vi "thermal_optical_camera_4.vi"() -> ()   [LabVIEW 2025]
uses:
  Global 1.vi
panel:
  in  "Stop (F)":bool
  in  "Acquisition Control:\nExposure Time [100, 3E7]":dbl=999.0 caption="Acquisition Control::Exposure Time" min=100.0 max=29999995.0
  in  "Analog Control:\nGain [0, 27]":dbl caption="Analog Control::Gain" min=0.0 max=27.045663671679687
  in  "Analog Control:\nBlack Level [-5, 10]":dbl caption="Analog Control::Black Level" min=-5.0000011920928955 max=10.000002384185791
  in  "Analog Control:\nGamma [0.25, 4.00]":dbl=0.800048828125 caption="Analog Control::Gamma" min=0.25 max=4.0 step=0.05
  out "Optical camera":T1(plugin-control)
  in  "optical capture interval (s)":dbl
  in  "File Path":string="C:\\Digambar\\Metal_thin_wall\\Optical_images\\Optical_images"
  out "File Name Out":string
  out "Frames":i32
  in  "thermal capture interval (s)":dbl
  out "Thermal camera":T1(plugin-control)
  out "Output":string
  in  "Flag Button":bool
  in  "Stop & Save":bool
  in  "Stop Preview":bool
  in  "Focus":dbl(slide) scale=0.0..100.0
  in  "Record":bool
  # "(1) Run VI"
  # "(2) After thermal camera calibration message (in terminal), press START"
  # "(3) Stop & Save"
  # "Destination for Optical Images:"
  # "Begin Record\nTHERMAL & OPTICAL"
  # "(Enter \"28\")"
  # "change folder names each time you run,\nso it saves data sets in dedicated folders:\nfolder1\nfolder2\nfolder3\netc..."
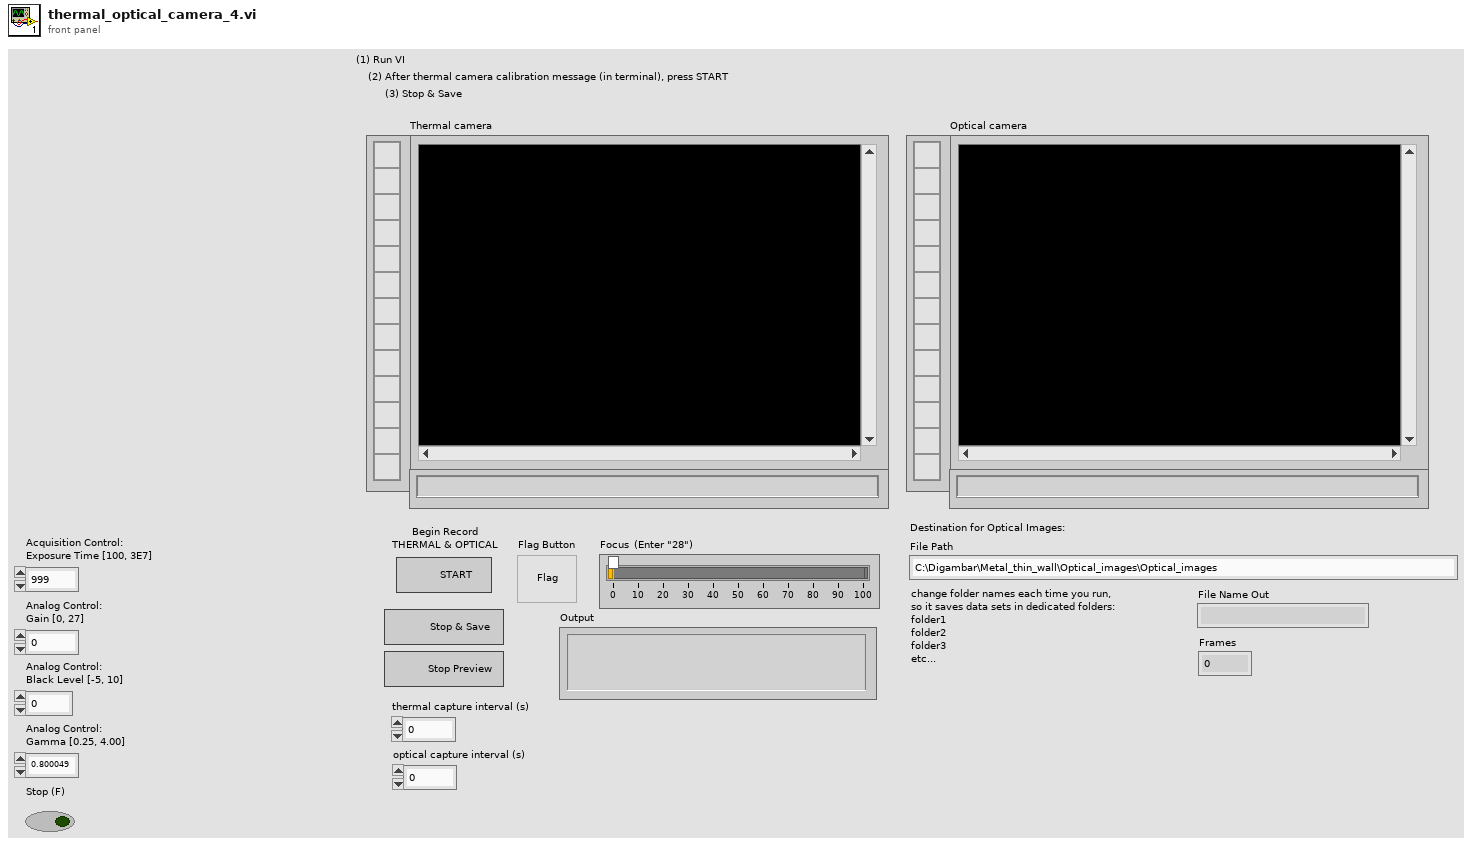
[diagram p1: front panel]
types:
  T1 = typedef "IMAQ Image.ctl" = refnum<image>
  T2 = enum16{"Standard", "Buffered", "CRLF", "Immediate"}
  T3 = enum16{"open", "replace", "create", "open or create", "replace or create", "replace or create with confirmation"}
  T4 = enum16{"big-endian, network order", "native, host order", "little-endian"}
  T5 = typedef "Image Type" = u32
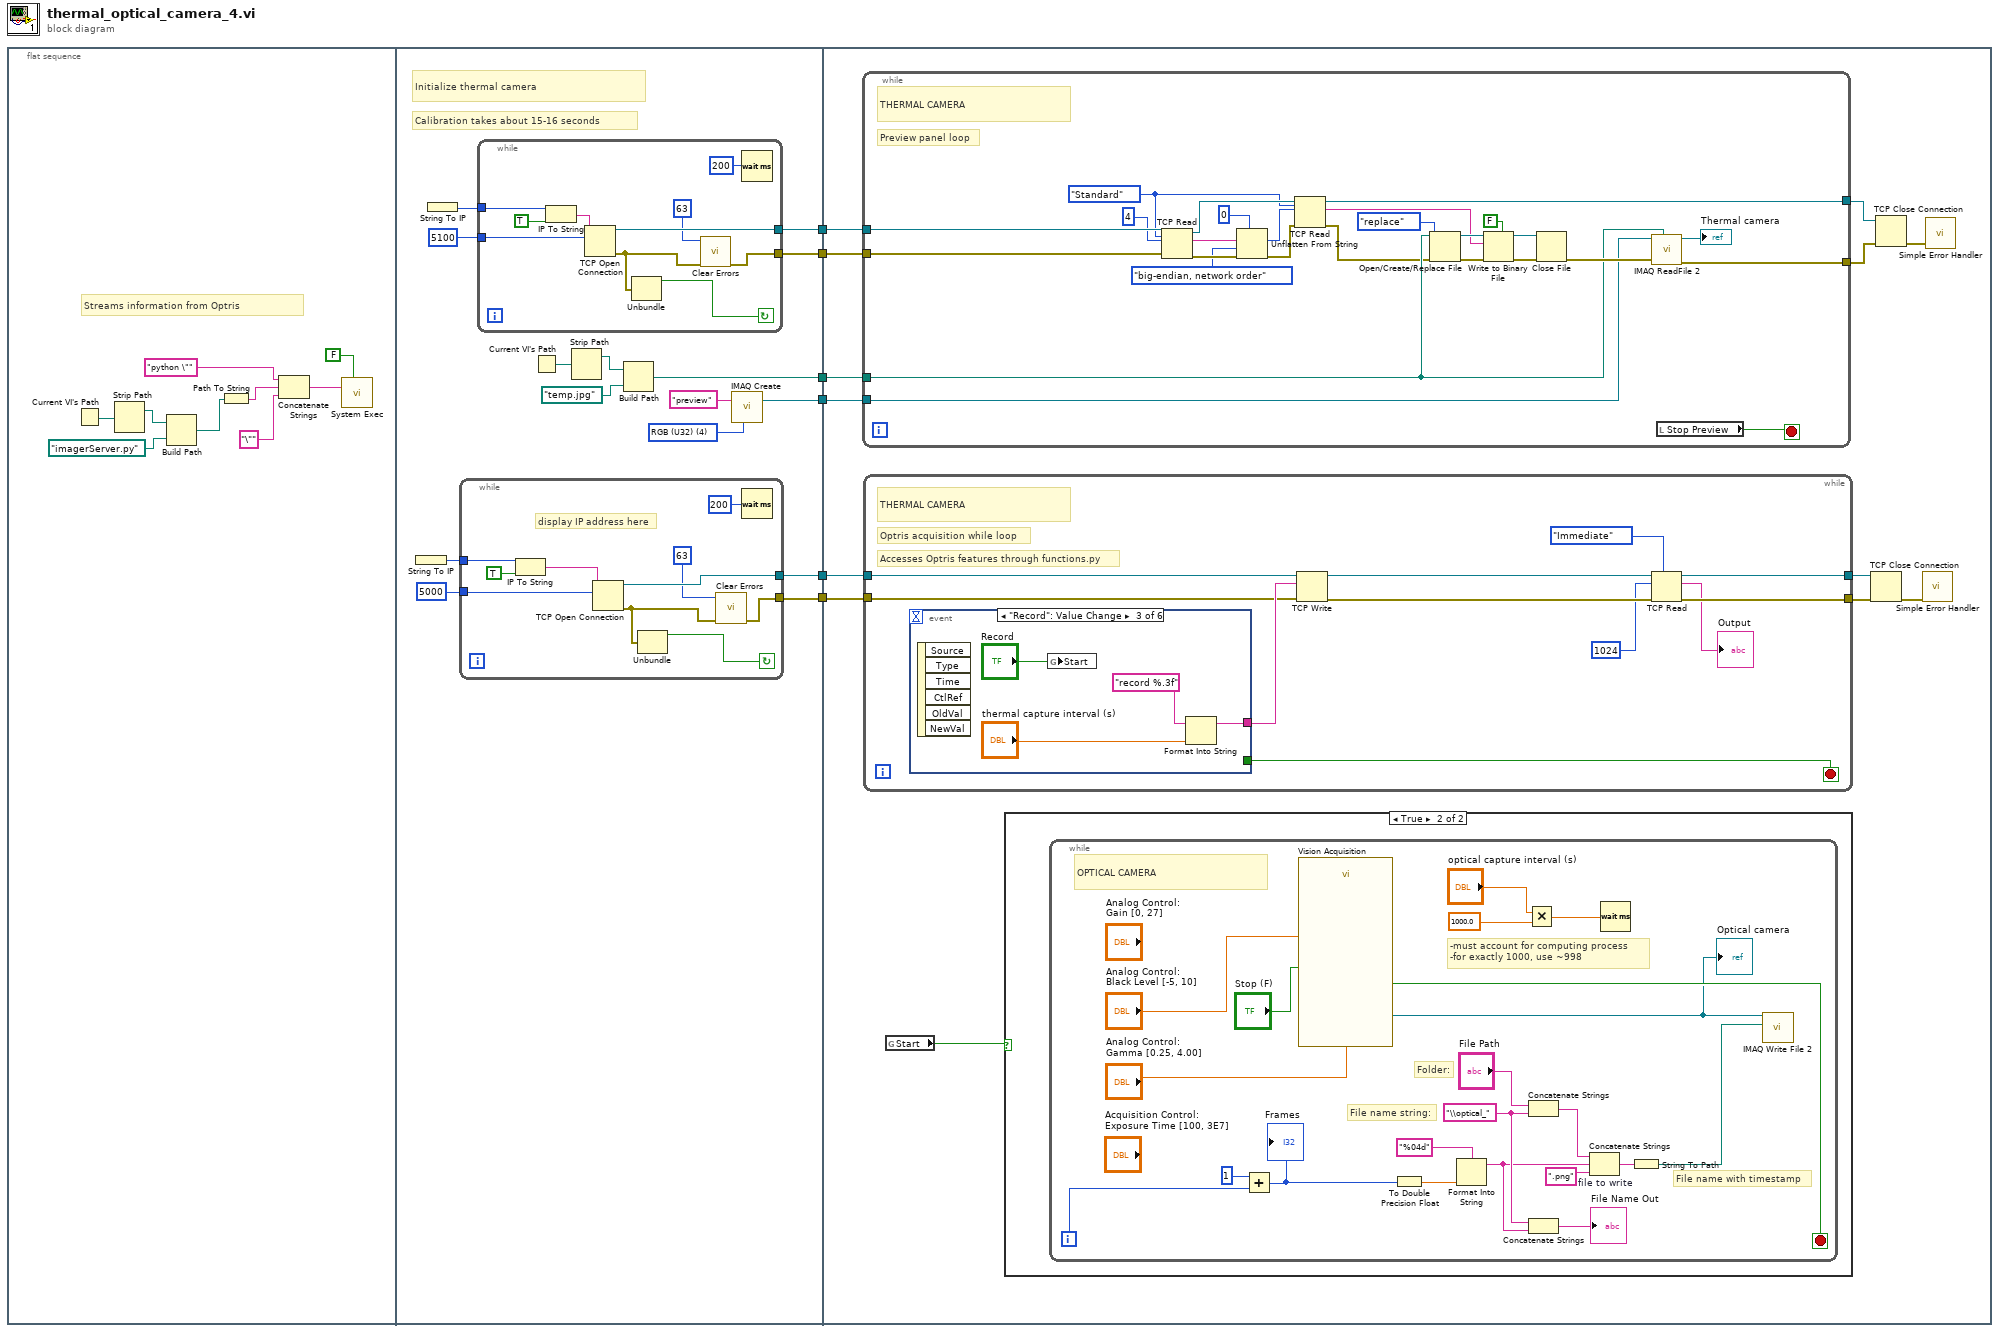
[diagram p0: block diagram]
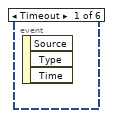
[diagram p3: hidden frame]
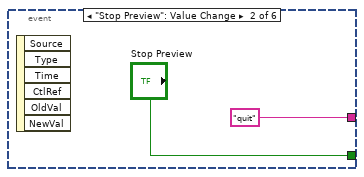
[diagram p4: hidden frame]
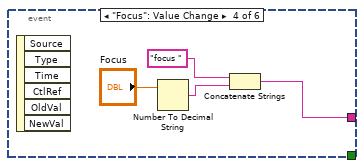
[diagram p5: hidden frame]
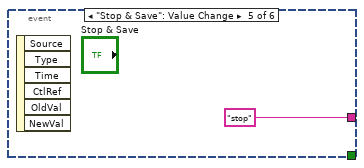
[diagram p6: hidden frame]
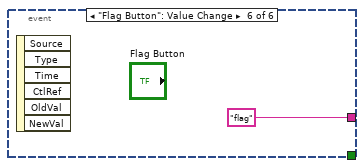
[diagram p7: hidden frame]
diagram:
  n1 = flat-sequence {
    tunnel: [w21] -> w6
    tunnel: [w20] -> w5
    tunnel: [w19] -> w4
    tunnel: [w18] -> w3
    tunnel: [w17] -> w2
    tunnel: [w16] -> w1
    tunnel: w1 -> [w57]
    tunnel: w2 -> [w58]
    tunnel: w3 -> [w53]
    tunnel: w4 -> [w52]
    tunnel: w5 -> [w59]
    tunnel: w6 -> [w60]
    frame #0 {
      # "Streams information from Optris"
      n2 = Current VI's Path() -> (path=w10:path)
      n3 = Strip Path(path=w10) -> (stripped path=w11:path)  [unwired: 1 out]
      n4 = Build Path(base path=w11, name or relative path=path "imagerServer.py") -> (appended path=w8:path)
      n5 = Path To String(path=w8) -> (string=w14:string)
      n6 = Concatenate Strings("python \"" ("string"), w14, "\"" ("string")) -> (w13:string)
      n7 = call <vilib>:"System Exec.vi"("wait until completion? (T)"=FALSE, "command line"=w13) -> ()  [unwired: 6 in, 4 out]
    }
    frame #1 {
      w22 = T5 4 items=["Grayscale (U8)", "Grayscale (I16)", "Grayscale (SGL)", "Complex (CSG)", "RGB (U32)", "HSL (U32)", "RGB (U64)", "Grayscale (U16)"] ("Image Type")
      # "Initialize thermal camera"
      # "Calibration takes about 15-16 seconds"
      n8 = String To IP() -> (0:w29:u32)  [unwired: 1 in]
      n9 = String To IP() -> (0:w30:u32)  [unwired: 1 in]
      n10 = while {
        tunnel: [w44] -> w19
        tunnel: [w50] -> w18
        tunnel: w29 -> [w48]
        tunnel: u16 5000 ("remote port or service name") -> [w46]
        stop <- w41 continue-if-true
        # "display IP address here"
        n11 = IP To String(1:TRUE ("dot notation? (F)"), 2:w48) -> (0:w49:string)
        n12 = TCP Open Connection(address=w49, remote port or service name=w46) -> (connection ID=w50:refnum<k5>, error out=w45:errorcluster)  [unwired: 3 in]
        n13 = Unbundle(w45) -> ("status"=w41:bool)  [unwired: 2 out]
        n14 = call <vilib>:"Clear Errors.vi"("error in (no error)"=w45, "specific error code to clear (0: all)"=63) -> ("error out"=w44:errorcluster)  [unwired: 4 in, 1 out]
        n15 = Wait (ms)(milliseconds to wait=u32 200) -> ()  [unwired: 1 out]
      }
      n16 = while {
        tunnel: w30 -> [w40]
        tunnel: [w34] -> w21
        tunnel: [w38] -> w20
        tunnel: u16 5100 ("remote port or service name") -> [w36]
        stop <- w31 continue-if-true
        n17 = IP To String(1:TRUE ("dot notation? (F)"), 2:w40) -> (0:w39:string)
        n18 = TCP Open Connection(address=w39, remote port or service name=w36) -> (connection ID=w38:refnum<k5>, error out=w35:errorcluster)  [unwired: 3 in]
        n19 = Unbundle(w35) -> ("status"=w31:bool)  [unwired: 2 out]
        n20 = call <vilib>:"Clear Errors.vi"("error in (no error)"=w35, "specific error code to clear (0: all)"=63) -> ("error out"=w34:errorcluster)  [unwired: 4 in, 1 out]
        n21 = Wait (ms)(milliseconds to wait=u32 200) -> ()  [unwired: 1 out]
      }
      n22 = Current VI's Path() -> (path=w28:path)
      n23 = Strip Path(path=w28) -> (stripped path=w27:path)  [unwired: 1 out]
      n24 = Build Path(base path=w27, name or relative path=path "temp.jpg") -> (appended path=w17:path)
      n25 = call "IMAQ Create"("Image Name"="preview", "Image Type"=w22) -> ("New Image"=w16:T1)  [unwired: 3 in, 1 out]
    }
    frame #2 {
      n26 = while {
        tunnel: [w131] -> w62
        tunnel: [w133] -> w63
        tunnel: w60 -> [w128]
        tunnel: w59 -> [w127]
        tunnel: w58 -> [w130]
        tunnel: w57 -> [w126]
        stop <- w129 stop-if-true
        w118 = T2."Standard" ("mode (standard)")
        # "THERMAL CAMERA"
        # "Preview panel loop"
        n27 = TCP Read(connection ID=w127, bytes to read=4, error in (no error)=w128, 7:w118) -> (connection ID out=w121:refnum<k5>, data out=w109:string, error out=w124:errorcluster)  [unwired: 1 in]
        n28 = Unflatten From String(type=0, binary string=w109, byte order (0:big-endian, network order)=T4."big-endian, network order", error in (no error)=w124) -> (value=w119:i32, error out=w120:errorcluster)  [unwired: 1 in, 1 out]
        n29 = TCP Read(connection ID=w121, bytes to read=w119, error in (no error)=w120, 7:w118) -> (connection ID out=w133:refnum<k5>, data out=w114:string, error out=w116:errorcluster)  [unwired: 1 in]
        n30 = Open/Create/Replace File(file path (use dialog)=w130, error in=w116, operation (0:open)=T3."replace") -> (refnum out=w115:refnum<file>, error out=w112:errorcluster)  [unwired: 3 in, 1 out]
        n31 = Write to Binary File(file (use dialog)=w115, data=w114, error in=w112, 5:FALSE ("prepend array or string size? (T)")) -> (refnum out=w110:refnum<file>, error out=w111:errorcluster)  [unwired: 2 in, 1 out]
        n32 = Close File(refnum=w110, error in=w111) -> (error out=w132:errorcluster)  [unwired: 1 out]
        n33 = call "IMAQ ReadFile 2"("File Path"=w130, "error in (no error)"=w132, "Image"=w126) -> ("error out"=w131:errorcluster, "Image Out"=→"Thermal camera":T1)  [unwired: 4 in, 3 out]
        n34 = local read "Stop Preview"() -> (w129:bool)
      }
      n35 = while {
        tunnel: [w94] -> w54
        tunnel: [w92] -> w55
        tunnel: w53 -> [w86]
        tunnel: w52 -> [w85]
        stop <- w87 stop-if-true
        # "THERMAL CAMERA"
        # "Optris acquisition while loop"
        # "Accesses Optris features through functions.py"
        n36 = event shown="[2] \"Record\": Value Change" {
          selector: _ -> [_ _ _ _ _ _]
          dyn-events: _ -> [_ _ _ _ _ _]
          timeout: _ -> [_ _ _ _ _ _]
          tunnel: [_ "quit" w101 w103 "stop" "flag"] -> w91
          tunnel: [_ "Stop Preview" _ _ _ _] -> w87
          event Timeout {
            n37 = event-data() -> ()  [unwired: 1 in, 3 out]
          }
          event "Stop Preview": Value Change {
            n38 = event-data() -> ()  [unwired: 1 in, 6 out]
          }
          event "Record": Value Change {
            n39 = event-data() -> ()  [unwired: 1 in, 6 out]
            n40 = global write "Global 1.vi" "Start"("Record") -> ()
            n41 = Format Into String(format string="record %.3f", "thermal capture interval (s)") -> (resulting string=w101:string)  [unwired: 2 in, 1 out]
          }
          event "Focus": Value Change {
            n42 = event-data() -> ()  [unwired: 1 in, 6 out]
            n43 = Number To Decimal String(number="Focus") -> (decimal integer string=w105:string)  [unwired: 1 in]
            n44 = Concatenate Strings("focus ", w105) -> (w103:string)
          }
          event "Stop & Save": Value Change {
            n45 = event-data() -> ()  [unwired: 1 in, 6 out]
          }
          event "Flag Button": Value Change {
            n46 = event-data() -> ()  [unwired: 1 in, 6 out]
          }
        }
        n47 = TCP Write(connection ID=w86, data in=w91, error in (no error)=w85) -> (connection ID out=w93:refnum<k5>, error out=w95:errorcluster)  [unwired: 1 in, 1 out]
        n48 = TCP Read(connection ID=w93, bytes to read=1024, error in (no error)=w95, 7:T2."Immediate" ("mode (standard)")) -> (connection ID out=w92:refnum<k5>, data out=→"Output":string, error out=w94:errorcluster)  [unwired: 1 in]
      }
      n49 = global read "Global 1.vi" "Start"() -> (w51:bool)
      n50 = case shown="True" w51 {
        frame False {
        }
        frame True {
          n51 = while {
            i -> [w65]
            stop <- w83 stop-if-true
            w71 = "\\optical_" ("string")
            # "-must account for computing process\n-for exactly 1000, use ~998"
            # "OPTICAL CAMERA"
            # "File name with timestamp"
            # "Folder:"
            # "File name string:"
            n52 = Add(x=1, y=w65) -> (x+y=w64:i32)
            "Frames" <- w64
            n53 = call "Vision Acquisition"("Analog Control::Black Level"="Analog Control:\nBlack Level [-5, 10]", "Analog Control::Gamma"="Analog Control:\nGamma [0.25, 4.00]", "Stop (F)"="Stop (F)") -> ("Image Out"=w82:T1, "Stopped"=w83:bool)  [unwired: 22 in, 1 out]
            "Optical camera" <- w82
            n54 = To Double Precision Float(number=w64) -> (double precision float=w67:dbl)
            n55 = Format Into String(format string="%04d" ("time format string (%c)"), w67) -> (resulting string=w69:string)  [unwired: 2 in, 1 out]
            n56 = Multiply(x="optical capture interval (s)", y=1000.0) -> (x*y=w77:dbl)
            n57 = Concatenate Strings("File Path", w71) -> (w72:string)
            n58 = Concatenate Strings(w71, w69) -> (→"File Name Out":string)
            n59 = Concatenate Strings "file to write"(w72, w69, ".png" ("string")) -> (w79:string)
            n60 = Wait (ms)(milliseconds to wait=w77) -> ()  [unwired: 1 out]
            n61 = String To Path(string=w79) -> (path=w75:path)
            n62 = call-poly "IMAQ Write File 2"("File Path"=w75, "Image"=w82) -> ()  [unwired: 8 in, 2 out]
          }
        }
      }
      n63 = TCP Close Connection(connection ID=w55, error in (no error)=w54) -> (error out=w56:errorcluster)  [unwired: 1 in, 1 out]
      n64 = TCP Close Connection(connection ID=w63, error in (no error)=w62) -> (error out=w61:errorcluster)  [unwired: 1 in, 1 out]
      n65 = call <vilib>:"Simple Error Handler.vi"("error in (no error)"=w56) -> ()  [unwired: 4 in, 5 out]
      n66 = call <vilib>:"Simple Error Handler.vi"("error in (no error)"=w61) -> ()  [unwired: 4 in, 5 out]
    }
  }
